vi "TMCM351-setPulsedivide.vi"(4 "错误输入":errorcluster caption="错误输入（无错误）", 5 "pulse_divid":i32=3, 7 "com in":refnum<visa-resource-name>) -> (0 "错误输出":errorcluster, 3 "com out":refnum<visa-resource-name>)   [LabVIEW 2018]
uses:
  module_param.vi
panel:
  # "设置分频"
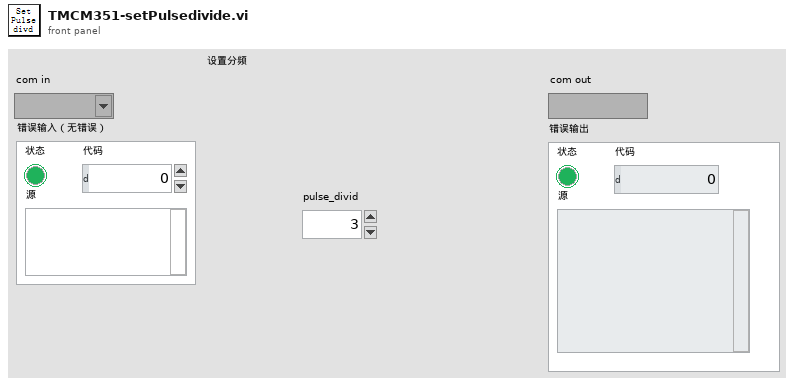
[diagram p1: front panel]
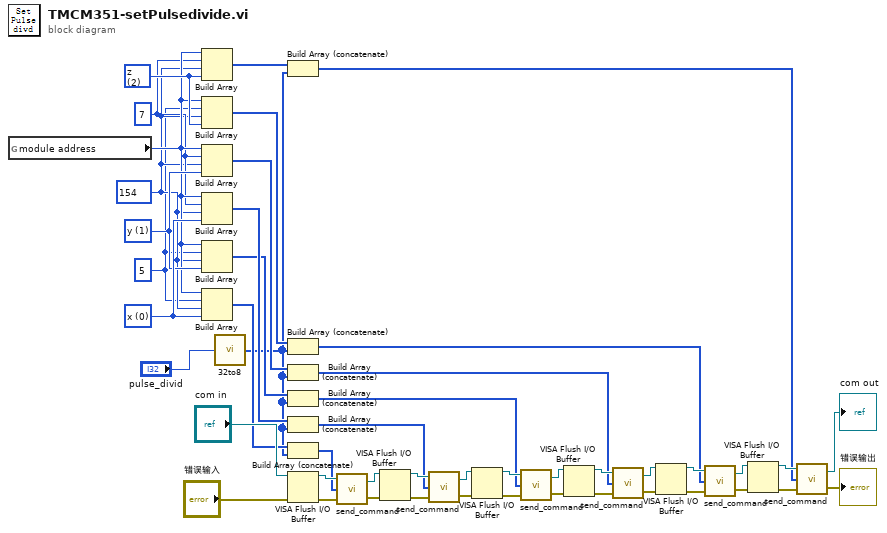
[diagram p0: block diagram]
diagram:
  w17 = u8 2 items=["x", "y", "z"] ("motor")
  w30 = u8 1 items=["x", "y", "z"] ("motor")
  w41 = u8 0 items=["x", "y", "z"] ("motor")
  w4 = u8 7 ("元素")
  w3 = u8 154
  w1 = u8 5
  n1 = global read "module_param.vi" "module address"() -> (w5:u8)
  n2 = Build Array(w5, w4, w3, w17) -> (w16:u8[])
  n3 = Build Array(w5, w1, w3, w17) -> (w19:u8[])
  n4 = Build Array(w5, w4, w3, w30) -> (w29:u8[])
  n5 = Build Array(w5, w4, w3, w41) -> (w40:u8[])
  n6 = Build Array(w5, w1, w3, w30) -> (w32:u8[])
  n7 = Build Array(w5, w1, w3, w41) -> (w43:u8[])
  n8 = call "32to8.vi"("32data_in"="pulse_divid") -> ("8Array"=w8:u8[])
  n9 = Build Array (concatenate)(w16, w8) -> (w11:u8[])
  n10 = Build Array (concatenate)(w19, w8) -> (w18:u8[])
  n11 = Build Array (concatenate)(w29, w8) -> (w24:u8[])
  n12 = Build Array (concatenate)(w32, w8) -> (w31:u8[])
  n13 = Build Array (concatenate)(w40, w8) -> (w35:u8[])
  n14 = Build Array (concatenate)(w43, w8) -> (w42:u8[])
  n15 = VISA Flush I/O Buffer(VISA resource name="com in", error in (no error)="错误输入") -> (VISA resource name out=w45:refnum<visa-resource-name>, error out=w44:errorcluster)  [unwired: 1 in]
  n16 = call "send_command.vi"("错误输入"=w44, 3:w42, "com in"=w45) -> ("错误输出"=w38:errorcluster, "com out"=w39:refnum<visa-resource-name>)
  n17 = VISA Flush I/O Buffer(VISA resource name=w39, error in (no error)=w38) -> (VISA resource name out=w37:refnum<visa-resource-name>, error out=w36:errorcluster)  [unwired: 1 in]
  n18 = call "send_command.vi"("错误输入"=w36, 3:w35, "com in"=w37) -> ("错误输出"=w22:errorcluster, "com out"=w23:refnum<visa-resource-name>)
  n19 = VISA Flush I/O Buffer(VISA resource name=w23, error in (no error)=w22) -> (VISA resource name out=w34:refnum<visa-resource-name>, error out=w33:errorcluster)  [unwired: 1 in]
  n20 = call "send_command.vi"("错误输入"=w33, 3:w31, "com in"=w34) -> ("错误输出"=w27:errorcluster, "com out"=w28:refnum<visa-resource-name>)
  n21 = VISA Flush I/O Buffer(VISA resource name=w28, error in (no error)=w27) -> (VISA resource name out=w26:refnum<visa-resource-name>, error out=w25:errorcluster)  [unwired: 1 in]
  n22 = call "send_command.vi"("错误输入"=w25, 3:w24, "com in"=w26) -> ("错误输出"=w9:errorcluster, "com out"=w10:refnum<visa-resource-name>)
  n23 = VISA Flush I/O Buffer(VISA resource name=w10, error in (no error)=w9) -> (VISA resource name out=w21:refnum<visa-resource-name>, error out=w20:errorcluster)  [unwired: 1 in]
  n24 = call "send_command.vi"("错误输入"=w20, 3:w18, "com in"=w21) -> ("错误输出"=w14:errorcluster, "com out"=w15:refnum<visa-resource-name>)
  n25 = VISA Flush I/O Buffer(VISA resource name=w15, error in (no error)=w14) -> (VISA resource name out=w13:refnum<visa-resource-name>, error out=w12:errorcluster)  [unwired: 1 in]
  n26 = call "send_command.vi"("错误输入"=w12, 3:w11, "com in"=w13) -> ("错误输出"=→"错误输出":errorcluster, "com out"=→"com out":refnum<visa-resource-name>)
